vi "Controller_Test.vi"() -> ()   [LabVIEW 2011, in "Controller Library.lvlib"]
uses:
  Controller Library.lvlib
  States/States.lvclass
  Non Linear PID Controller/Non Linear PID Controller.lvclass
  ROV/Vessel.lvclass
  <vilib>/Analysis/Matrix/Datatypes/RealMatrix.ctl
  <vilib>/Analysis/Matrix/NI_Matrix.lvlib
panel:
  in  "Thrust_max":dbl[](array[numeric])
  in  "D_NL":T1
  in  "D_L":T1
  in  "M_A":T1
  in  "M_RB":T1
  in  "K_anti":T1
  in  "Int_limit":dbl[](array[numeric])
  in  "acc_d":dbl[](array[numeric])
  in  "nu_d":dbl[](array[numeric])
  in  "dt":dbl
  in  "K_d":T1
  in  "K_i":T1
  in  "K_p":T1
  out "tau":dbl[](array[numeric])
  in  "nu":dbl[](array[numeric])
  in  "eta_d":dbl[](array[numeric])
  in  "eta":dbl[](array[numeric])
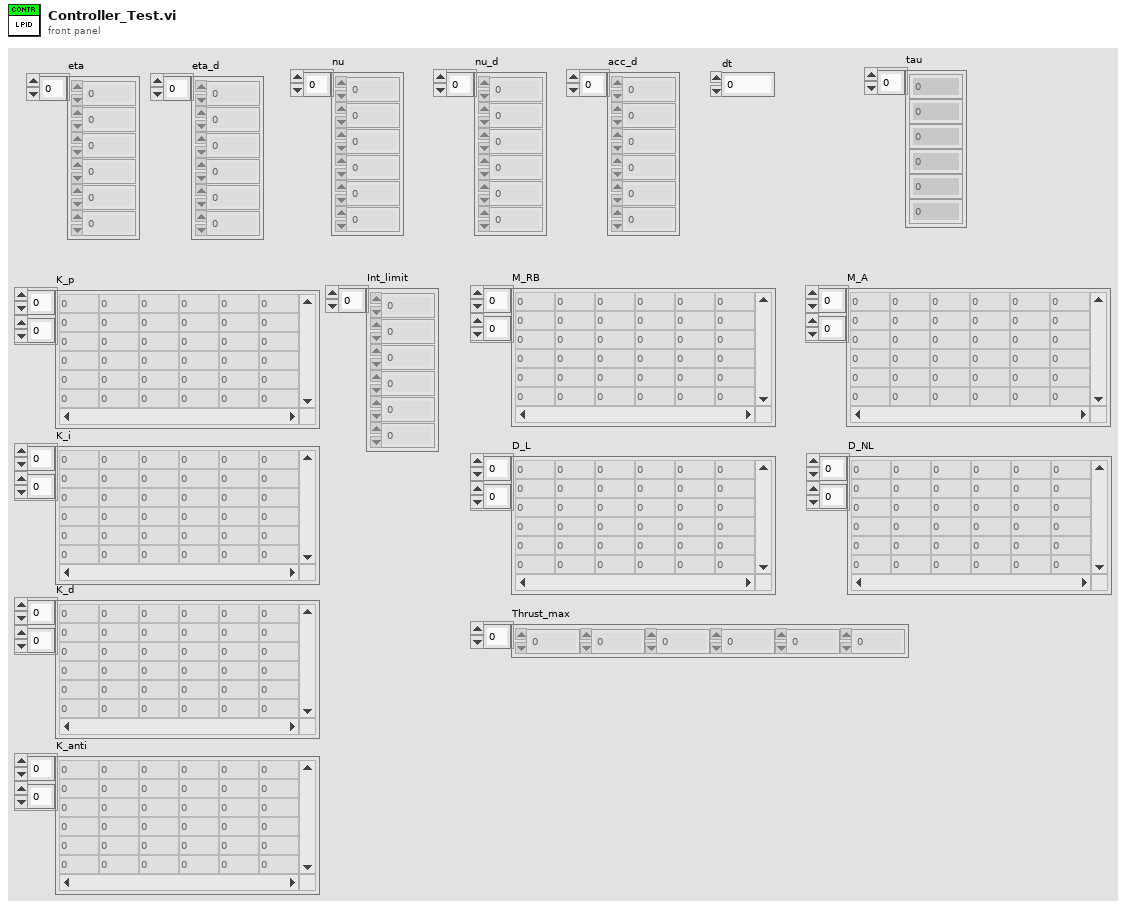
[diagram p1: front panel]
types:
  T1 = typedef "NI_Matrix.lvlib/RealMatrix.ctl" = dbl[][]
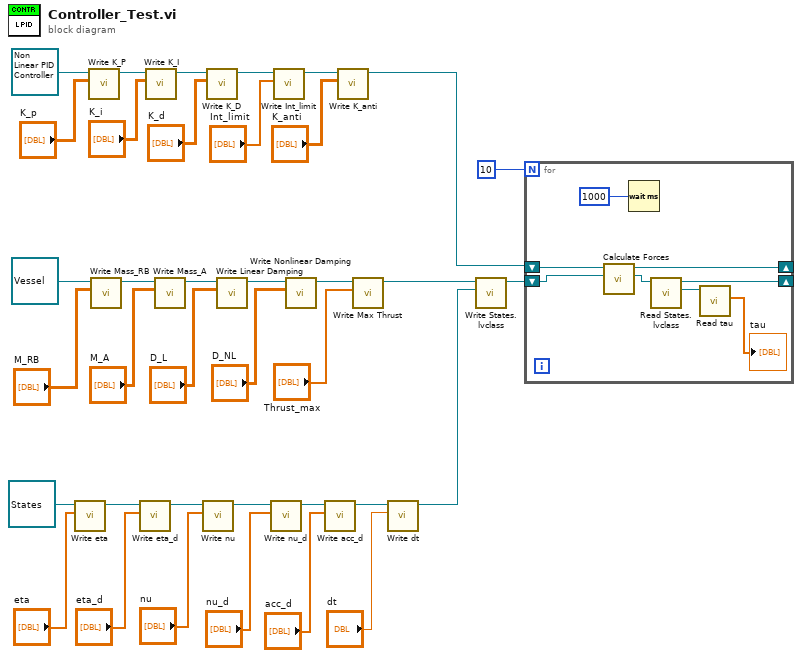
[diagram p0: block diagram]
diagram:
  n1 = call-dynamic "Write eta.vi"("eta"="eta", "States in"=refnum<class "States.lvclass"> refnum ("States.lvclass")) -> ("States out"=w33:refnum<class "States.lvclass">)  [unwired: 8 in, 1 out]
  n2 = call-dynamic "Write K_P.vi"("Real Matrix"="K_p", "PID Controller in"=refnum<class "Non Linear PID Controller.lvclass"> refnum ("Controller Library:Non Linear PID Controller.lvclass")) -> ("PID Controller out"=w31:refnum<class "Non Linear PID Controller.lvclass">)  [unwired: 8 in, 1 out]
  n3 = call "Write Mass_RB.vi"("Real Matrix"="M_RB", "Vessel in"=refnum<class "Vessel.lvclass"> refnum ("Vessel.lvclass")) -> ("Vessel out"=w10:refnum<class "Vessel.lvclass">)  [unwired: 8 in, 1 out]
  n4 = call-dynamic "Write eta_d.vi"("eta_d"="eta_d", "States in"=w33) -> ("States out"=w32:refnum<class "States.lvclass">)  [unwired: 8 in, 1 out]
  n5 = call-dynamic "Write K_I.vi"("Real Matrix"="K_i", "PID Controller in"=w31) -> ("PID Controller out"=w30:refnum<class "Non Linear PID Controller.lvclass">)  [unwired: 8 in, 1 out]
  n6 = call "Write Mass_A.vi"("Real Matrix"="M_A", "Vessel in"=w10) -> ("Vessel out"=w9:refnum<class "Vessel.lvclass">)  [unwired: 8 in, 1 out]
  n7 = call-dynamic "Write nu.vi"("nu"="nu", "States in"=w32) -> ("States out"=w24:refnum<class "States.lvclass">)  [unwired: 8 in, 1 out]
  n8 = call-dynamic "Write K_D.vi"("Real Matrix"="K_d", "PID Controller in"=w30) -> ("PID Controller out"=w16:refnum<class "Non Linear PID Controller.lvclass">)  [unwired: 8 in, 1 out]
  n9 = call "Write Linear Damping.vi"("Real Matrix"="D_L", "Vessel in"=w9) -> ("Vessel out"=w8:refnum<class "Vessel.lvclass">)  [unwired: 8 in, 1 out]
  n10 = call-dynamic "Write nu_d.vi"("nu_d"="nu_d", "States in"=w24) -> ("States out"=w23:refnum<class "States.lvclass">)  [unwired: 8 in, 1 out]
  n11 = call-dynamic "Write Int_limit.vi"("Int_limit"="Int_limit", "Non Linear PID Controller in"=w16) -> ("Non Linear PID Controller out"=w15:refnum<class "Non Linear PID Controller.lvclass">)  [unwired: 8 in, 1 out]
  n12 = call "Write Nonlinear Damping.vi"("Real Matrix"="D_NL", "Vessel in"=w8) -> ("Vessel out"=w7:refnum<class "Vessel.lvclass">)  [unwired: 8 in, 1 out]
  n13 = call "Write acc_d.vi"("acc_d"="acc_d", "States in"=w23) -> ("States out"=w22:refnum<class "States.lvclass">)  [unwired: 8 in, 1 out]
  n14 = call-dynamic "Write K_anti.vi"("Real Matrix"="K_anti", "Non Linear PID Controller in"=w15) -> ("Non Linear PID Controller out"=w14:refnum<class "Non Linear PID Controller.lvclass">)  [unwired: 8 in, 1 out]
  n15 = call "Write Max Thrust.vi"("Max Thrust"="Thrust_max", "Vessel in"=w7) -> ("Vessel out"=w6:refnum<class "Vessel.lvclass">)  [unwired: 8 in, 1 out]
  n16 = call-dynamic "Write dt.vi"("dt"="dt", "States in"=w22) -> ("States out"=w18:refnum<class "States.lvclass">)  [unwired: 8 in, 1 out]
  n17 = call "Write States.lvclass.vi"("States.lvclass"=w18, "Vessel in"=w6) -> ("Vessel out"=w17:refnum<class "Vessel.lvclass">)  [unwired: 8 in, 1 out]
  n18 = for {
    N: 10 -> [_]
    shift-right: [w44] -> _
    shift-left: w14 -> [w45]
    shift-right: [w39] -> _
    shift-left: w17 -> [w38]
    n19 = call-dynamic "Calculate Forces.vi"("Vessel in"=w38, "Non Linear PID Controller in"=w45) -> ("Vessel out"=w41:refnum<class "Vessel.lvclass">, "Non Linear PID Controller out"=w44:refnum<class "Non Linear PID Controller.lvclass">)  [unwired: 7 in, 1 out]
    n20 = Wait (ms)(milliseconds to wait=1000) -> ()  [unwired: 1 out]
    n21 = call "Read States.lvclass.vi"("Vessel in"=w41) -> ("States.lvclass"=w40:refnum<class "States.lvclass">, "Vessel out"=w39:refnum<class "Vessel.lvclass">)  [unwired: 8 in, 1 out]
    n22 = call-dynamic "Read tau.vi"("States in"=w40) -> ("tau"=→"tau":dbl[])  [unwired: 8 in, 2 out]
  }
